vi "Post_Pelletron_Tick.vi"(7 "error in (no error)":errorcluster, 10 "Input data":T1) -> (0 "error out":errorcluster)   [LabVIEW 2013]
uses:
  PelletronLabview.ctl
  Private/Controls/Pelletron.ctl
panel:
  out "Front Panel Window:Open":bool
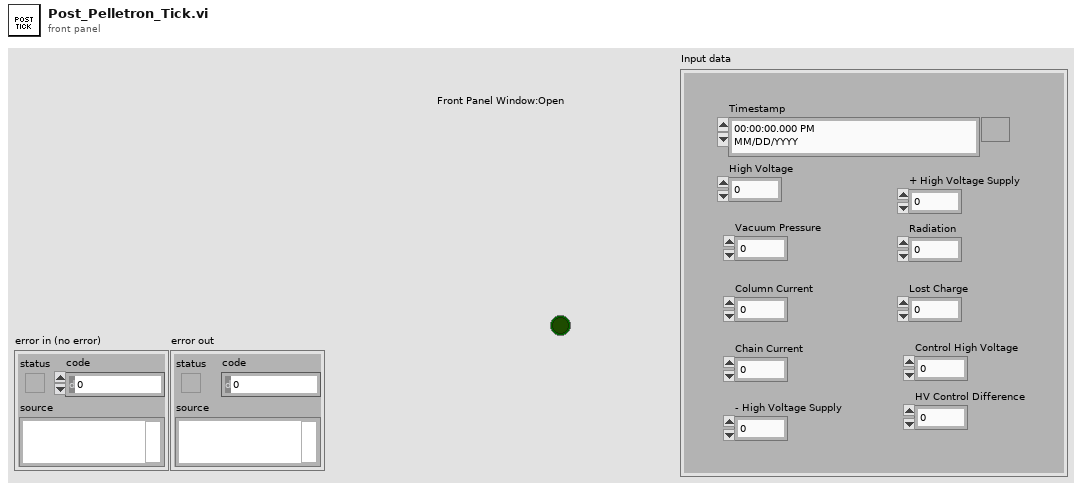
[diagram p1: front panel]
types:
  T1 = typedef "PelletronLabview.ctl" = cluster{"Timestamp":timestamp, "High Voltage":sgl, "+ High Voltage Supply":dbl, "- High Voltage Supply":dbl, "HV Control Difference":dbl, "Vacuum Pressure":sgl, "Radiation":dbl, "Column Current":sgl, "Lost Charge":dbl, "Chain Current":sgl, "Control High Voltage":dbl}
  T2 = enum32{"Bad", "Idle", "Run top level", "Running"}
  T3 = typedef "Pelletron.ctl" = cluster{"ID":i32, "Integer Timestamp":u64, "High Voltage":sgl, "+ High Voltage Supply":sgl, "- High Voltage Supply":sgl, "HV Control Difference":sgl, "Vacuum Pressure":sgl, "Radiation":sgl, "Column Current":sgl, "Lost Charge":sgl, "Chain Current":sgl, "Control High Voltage":sgl}
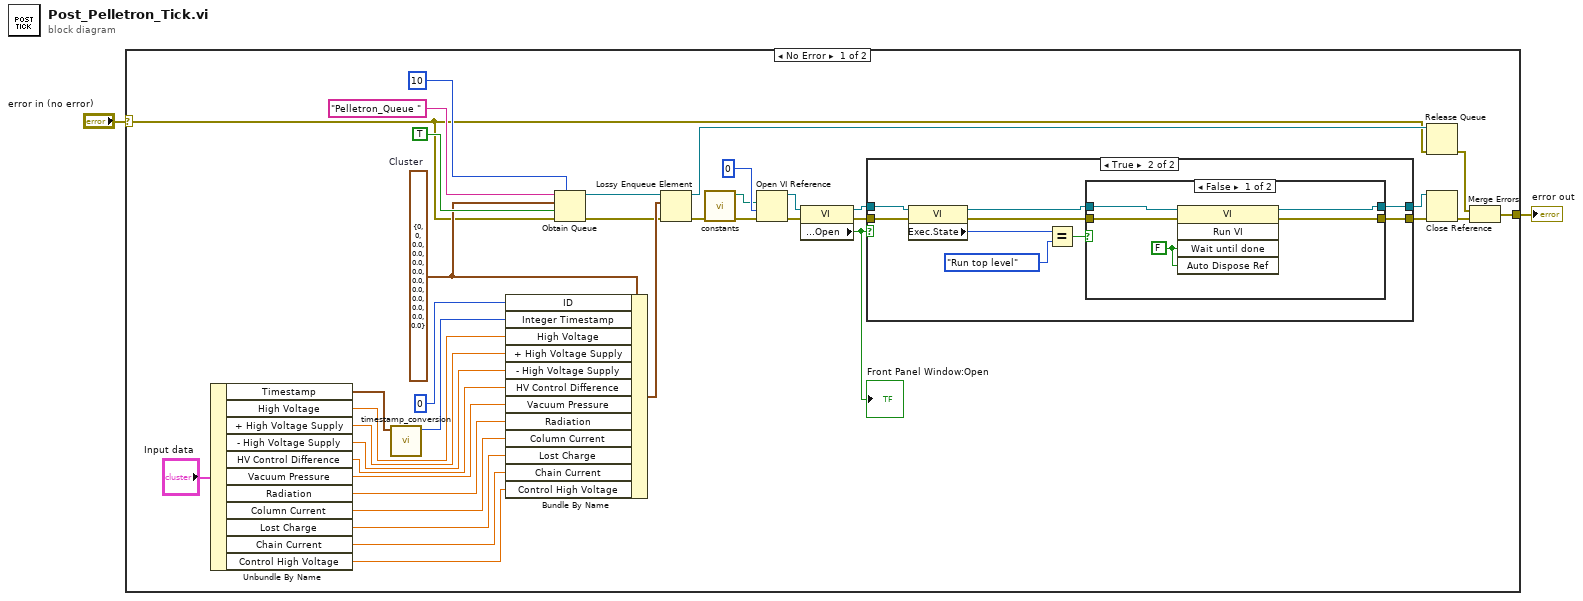
[diagram p0: block diagram]
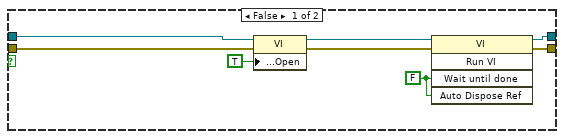
[diagram p2: hidden frame]
diagram:
  n1 = case shown="No Error" "error in (no error)" {
    selector: "error in (no error)" -> [w3 w64]
    tunnel: [w14 w64] -> w1
    frame No Error {
      w32 = T3 {"ID"=0, "Integer Timestamp"=0, "High Voltage"=0.0, "+ High Voltage Supply"=0.0, "- High Voltage Supply"=0.0, "HV Control Difference"=0.0, "Vacuum Pressure"=0.0, "Radiation"=0.0, "Column Current"=0.0, "Lost Charge"=0.0, "Chain Current"=0.0, "Control High Voltage"=0.0}  # Cluster
      n2 = Unbundle By Name("Input data") -> ("Timestamp"=w28:timestamp, "High Voltage"=w27:sgl, "+ High Voltage Supply"=w26:dbl, "- High Voltage Supply"=w25:dbl, "HV Control Difference"=w24:dbl, "Vacuum Pressure"=w23:sgl, "Radiation"=w22:dbl, "Column Current"=w21:sgl, "Lost Charge"=w20:dbl, "Chain Current"=w19:sgl, "Control High Voltage"=w18:dbl)
      n3 = call "timestamp_conversion.vi"("Time Stamp"=w28) -> ("Integer Time"=w31:i64)  [unwired: 8 in, 1 out]
      n4 = Bundle By Name(cluster=w32, "ID"=0, "Integer Timestamp"=w31, "High Voltage"=w27, "+ High Voltage Supply"=w26, "- High Voltage Supply"=w25, "HV Control Difference"=w24, "Vacuum Pressure"=w23, "Radiation"=w22, "Column Current"=w21, "Lost Charge"=w20, "Chain Current"=w19, "Control High Voltage"=w18) -> (w30:T3)
      n5 = Obtain Queue(max queue size (-1, unlimited)=10, name (unnamed)="Pelletron_Queue ", element data type=w32, create if not found? (T)=TRUE, error in (no error)=w3) -> (queue out=w39:refnum<queue>, error out=w15:errorcluster)  [unwired: 1 out]
      n6 = Lossy Enqueue Element(queue=w39, element=w30, error in (no error)=w15) -> (queue out=w17:refnum<queue>, error out=w11:errorcluster)  [unwired: 2 out]
      n7 = call "constants.vi"("error in (no error)"=w11) -> ("error out"=w10:errorcluster, "DB connection File Path"=w12:path)  [unwired: 4 in, 5 out]
      n8 = Open VI Reference(vi path=w12, options=0, error in (no error)=w10) -> (vi reference=w36:refnum<vi>, error out=w37:errorcluster)  [unwired: 3 in]
      n9 = property class="VI"(reference=w36, error in=w37) -> (reference out=w7:refnum<vi>, error out=w6:errorcluster, "Front Panel.Open"=w8:bool)
      "Front Panel Window:Open" <- w8
      n10 = case shown="True" w8 {
        tunnel: w6 -> [w47 w55]
        tunnel: [w43 w48] -> w4
        tunnel: w7 -> [w42 w56]
        tunnel: [w44 w49] -> w5
        frame False {
          w40 = FALSE ("Wait Until Done")
          n11 = property class="VI"(reference=w42, error in=w47, "Front Panel.Open"=TRUE ("Front Panel Window:Open")) -> (reference out=w46:refnum<vi>, error out=w45:errorcluster)
          n12 = invoke class="VI" method="Run VI"(reference=w46, error in=w45, "Wait until done"=w40, "Auto Dispose Ref"=w40) -> (reference out=w44:refnum<vi>, error out=w43:errorcluster)  [unwired: 1 in, 3 out]
        }
        frame True {
          n13 = property class="VI"(reference=w56, error in=w55) -> (reference out=w51:refnum<vi>, error out=w50:errorcluster, "Exec.State"=w54:T2)
          n14 = Equal?(x=w54, y=T2."Run top level" ("Execution:State 2")) -> (x = y?=w52:bool)
          n15 = case shown="False" w52 {
            tunnel: w51 -> [w60 w63]
            tunnel: w50 -> [w59 w62]
            tunnel: [w58 w63] -> w49
            tunnel: [w57 w62] -> w48
            frame False {
              w61 = FALSE ("Wait Until Done")
              n16 = invoke class="VI" method="Run VI"(reference=w60, error in=w59, "Wait until done"=w61, "Auto Dispose Ref"=w61) -> (reference out=w58:refnum<vi>, error out=w57:errorcluster)  [unwired: 1 in, 3 out]
            }
            frame True {
            }
          }
        }
      }
      n17 = Release Queue(queue=w17, error in (no error)=w3) -> (error out=w16:errorcluster)  [unwired: 1 in, 2 out]
      n18 = Close Reference(reference=w5, error in (no error)=w4) -> (error out=w13:errorcluster)
      n19 = Merge Errors(w16, w13) -> (w14:errorcluster)
    }
    frame Error {
    }
  }
  "error out" <- w1
